vi "motorstepper.vi"() -> ()   [LabVIEW 2019]
uses:
  <vilib>/eio/EIONode/EIONode.xnode
  <vilib>/rvi/eio/common/nirviEmuTemplateMethod_errors.vi
panel:
  in  "Count(Ticks)":u32
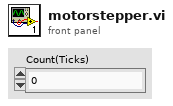
[diagram p1: front panel]
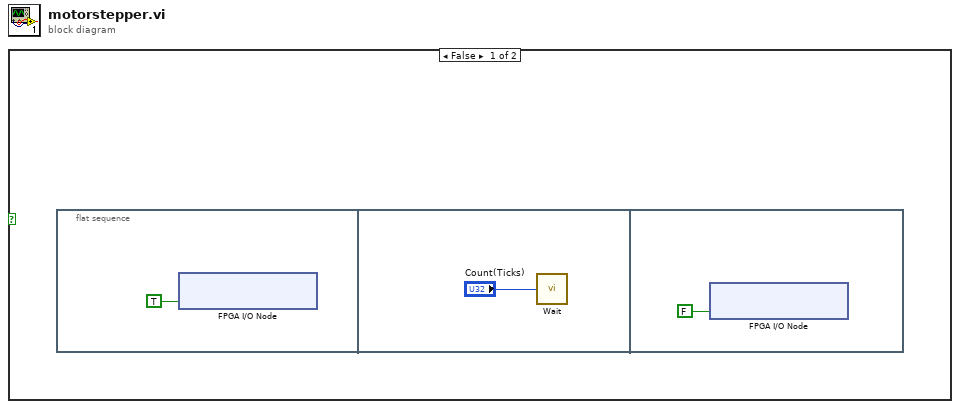
[diagram p0: block diagram]
diagram:
  n1 = case shown="False" {
    selector: _ -> [_ _]
    frame False {
      n2 = flat-sequence {
        frame #0 {
          n3 = xnode "FPGA I/O Node"("ConnectorA/DIO0"=TRUE) -> ()  [unwired: 1 in, 1 out]
        }
        frame #1 {
          n4 = call "Wait"("Count(Ticks)"="Count(Ticks)") -> ()  [unwired: 1 out]
        }
        frame #2 {
          n5 = xnode "FPGA I/O Node"("ConnectorA/DIO0"=FALSE) -> ()  [unwired: 1 in, 1 out]
        }
      }
    }
    frame True {
    }
  }
